vi "PlayWithSync_Third.vi"   [LabVIEW 2017]
uses:
  <vilib>/Waveform/DWDTOps.llb/DWDT Analog to Digital.vi
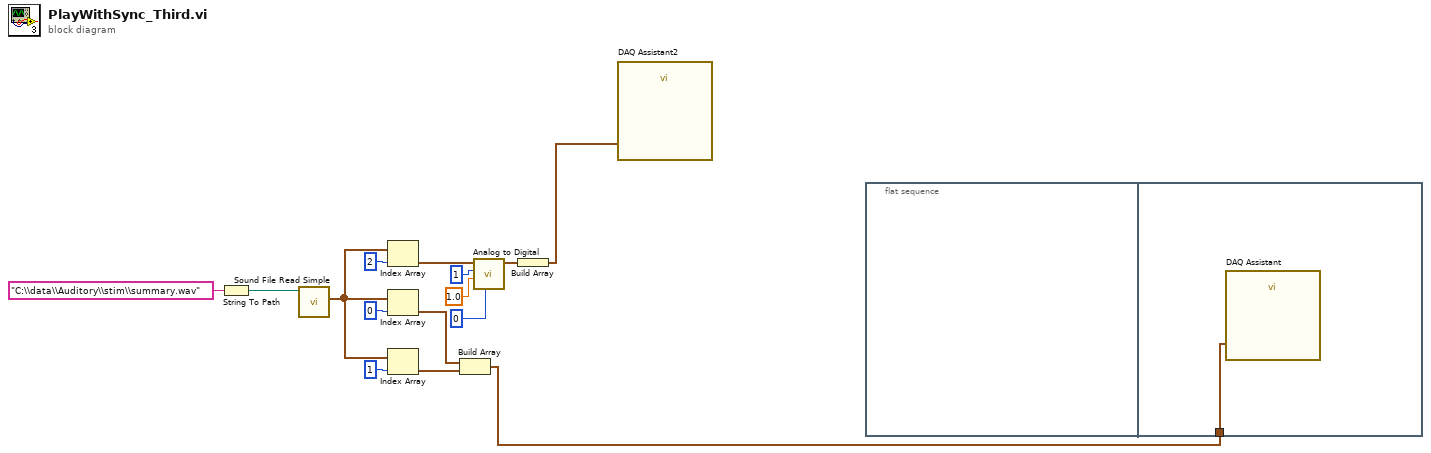
[diagram p0: block diagram]
diagram:
  n1 = String To Path(string="C:\\data\\Auditory\\stim\\summary.wav") -> (path=w15:path)
  n2 = call <vilib>:"Sound File Read Simple.vi"("path"=w15) -> ("data"=w10:waveform(dbl)[])  [unwired: 7 in, 3 out]
  n3 = Index Array(array=w10, index=2) -> (element=w4:waveform(dbl))
  n4 = Index Array(array=w10, index=0) -> (element=w3:waveform(dbl))
  n5 = Index Array(array=w10, index=1) -> (element=w9:waveform(dbl))
  n6 = Build Array(w3, w9) -> (w2:waveform(dbl)[])
  n7 = call-poly <vilib>:"Analog to Digital.vi"("data format (offset binary)"=0, "full-scale range (pk-pk)"=1.0, "resolution (16 bit)"=1, "analog waveform"=w4) -> ("digital waveform"=w5:digitalwaveform)  [unwired: 4 in, 3 out]
  n8 = Build Array(w5) -> (w1:digitalwaveform[])
  n9 = call "DAQ Assistant2"("data"=w1) -> ()  [unwired: 17 in, 2 out]
  n10 = flat-sequence {
    tunnel: w2 -> [w16]
    frame #0 {
    }
    frame #1 {
      n11 = call "DAQ Assistant"("data"=w16) -> ()  [unwired: 17 in, 2 out]
    }
  }
